vi "Pie Diagram.vi"(6 "Array":i32[](array[numeric]), 8 "error in (no error)":errorcluster, 9 "Chart Area Size":cluster{"Width":dbl, "Height":dbl}, 10 "Height":dbl, 11 "Values":dbl[](array[numeric])) -> (0 "error out":errorcluster, 3 "new picture":picture)   [LabVIEW 2019, in "Zen Analytics.lvlib" / "Zen Analytics.lvclass"]
uses:
  Zen Analytics.lvclass
panel:
  # "1) % of Pass Results\n2) % of Fail Results"
  # "Color"
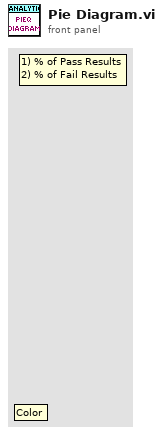
[diagram p1: front panel]
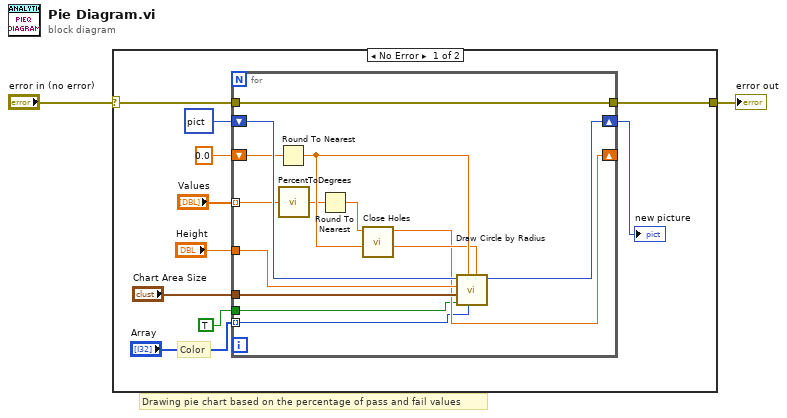
[diagram p0: block diagram]
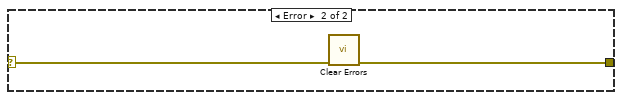
[diagram p2: hidden frame]
diagram:
  # "Drawing pie chart based on the percentage of pass and fail values"
  n1 = case shown="No Error" "error in (no error)" {
    selector: "error in (no error)" -> [w3 w28]
    tunnel: [w4 w27] -> w1
    frame No Error {
      # "Color"
      n2 = for {
        shift-right: [w15] -> w7
        shift-left: picture data[5B] ("new picture") -> [w26]
        tunnel: "Chart Area Size" -> [w24]
        tunnel: "Height" -> [w25]
        shift-right: [w19] -> _
        shift-left: 0.0 -> [w23]
        tunnel: TRUE ("fill?(F)") -> [w17]
        tunnel: "Array" -> [w16] mode=indexing
        tunnel: "Values" -> [w14] mode=indexing
        tunnel: [w13] -> w4
        tunnel: w3 -> [w13]
        n3 = Round To Nearest(number=w23) -> (nearest integer value=w22:dbl)
        n4 = call "PercentToDegrees.vi"("Percent"=w14) -> ("Degrees"=w21:dbl)
        n5 = Round To Nearest(number=w21) -> (nearest integer value=w18:dbl)
        n6 = call "Close Holes.vi"("Start Angle"=w22, "Preliminary Arc Size"=w18) -> ("Final Arc Size"=w20:dbl, "Final Angle"=w19:dbl)  [unwired: 8 out]
        n7 = call <vilib>:"Draw Circle by Radius.vi"("arc size(360)"=w20, "color(black)"=w16, "start angle(0)"=w22, "fill?(F)"=w17, "pixel center"=w24, "radius"=w25, "picture"=w26) -> ("new picture"=w15:picture)  [unwired: 1 in, 3 out]
      }
      "new picture" <- w7
    }
    frame Error {
      n8 = call <vilib>:"Clear Errors.vi"("error in (no error)"=w28) -> ("error out"=w27:errorcluster)  [unwired: 5 in, 1 out]
    }
  }
  "error out" <- w1
